vi "ultrasonic (SubVI).vi"(11 "[ESC] in":bool) -> (1 "Boolean":bool, 2 "range [centimeters] 2":sgl(slide) scale=0.0..80.0, 3 "range finder output 2":string, 4 "0, 1":i16)   [LabVIEW 2021]
uses:
  <vilib>/Instr/_visa.llb/VISA Configure Serial Port (Instr).vi
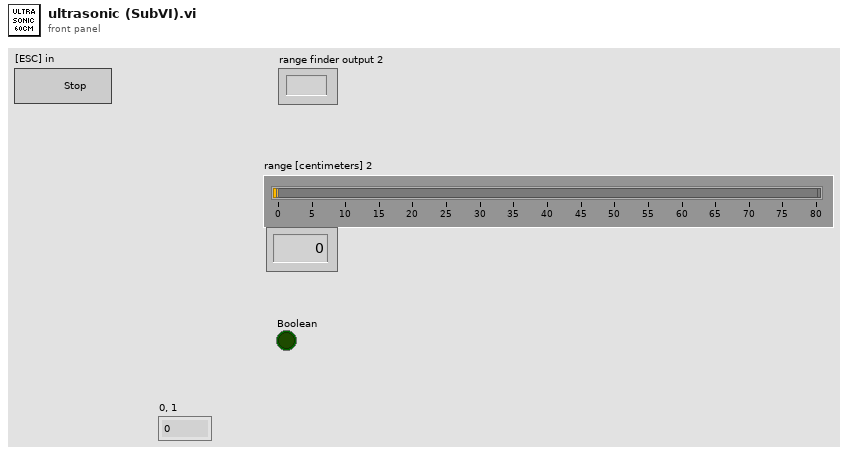
[diagram p1: front panel]
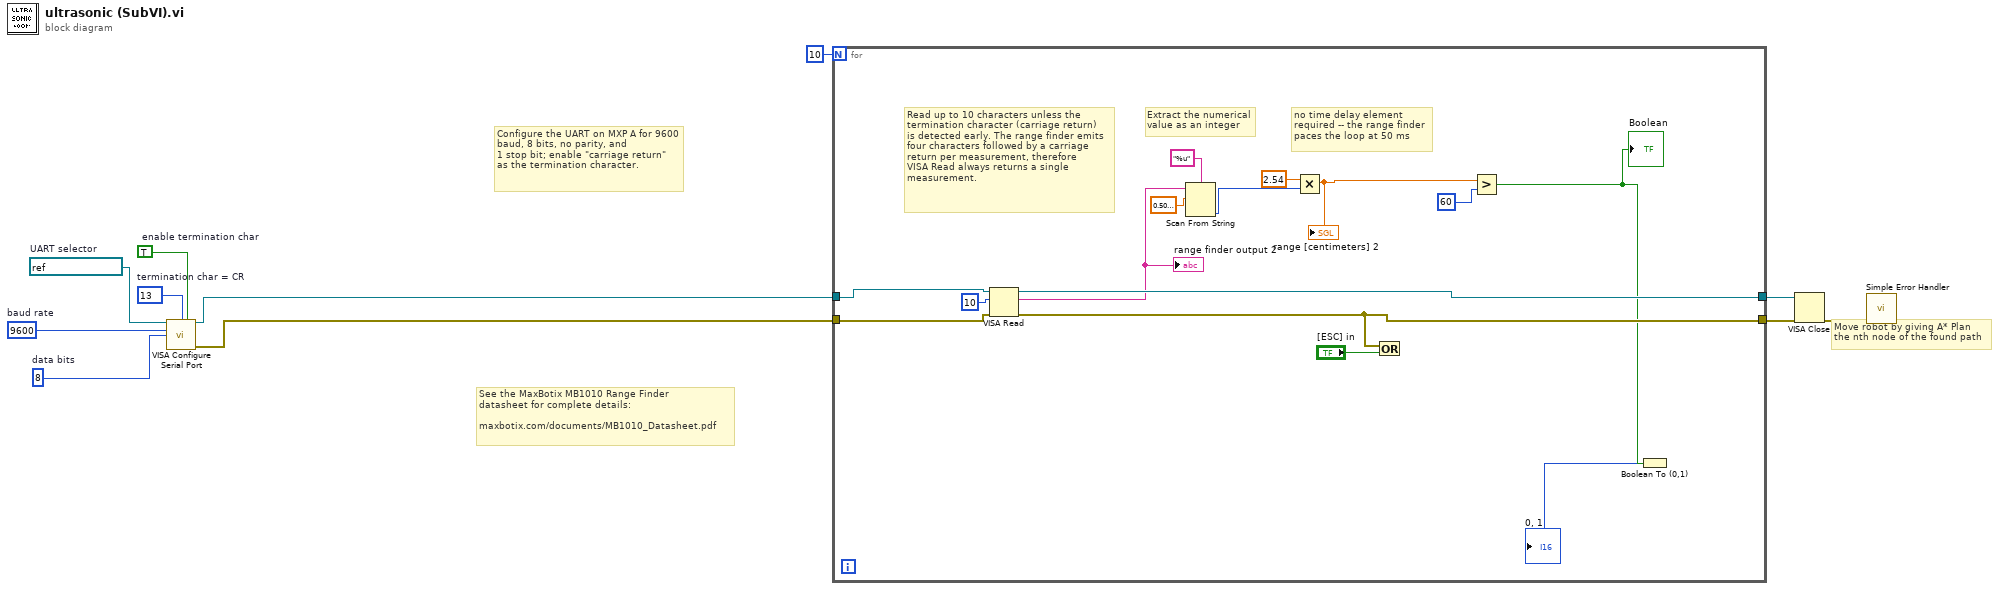
[diagram p0: block diagram]
diagram:
  w4 = u16 8  # data bits
  w5 = u32 9600  # baud rate
  w8 = refnum<visa-resource-name> "ASRL1::INSTR"  # UART selector
  w7 = u8 13  # termination char = CR
  w6 = TRUE  # enable termination char
  # "See the MaxBotix MB1010 Range Finder\ndatasheet for complete details:\n\nmaxbotix.com/documents/MB1010_Datasheet.pdf"
  # "Configure the UART on MXP A for 9600 baud, 8 bits, no parity, and\n1 stop bit; enable \"carriage return\"\nas the termination character."
  # "Move robot by giving A* Plan\nthe nth node of the found path"
  n1 = call-poly "VISA Configure Serial Port"("VISA resource name"=w8, "termination char\n(0xA = '\\n' = LF)"=w7, "Enable Termination\nChar (T)"=w6, "baud rate (9600)"=w5, "data bits (8)"=w4) -> ("VISA resource name out"=w3:refnum<visa-resource-name>, "error out"=w2:errorcluster)  [unwired: 9 in]
  n2 = for {
    N: 10 -> [_]
    tunnel: w3 -> [w24]
    tunnel: [w25] -> w9
    tunnel: w2 -> [w23]
    tunnel: [w26] -> w10
    # "Read up to 10 characters unless the \ntermination character (carriage return)\nis detected early. The range finder emits\nfour characters followed by a carriage\nreturn per measurement, therefore\nVISA Read always returns a single measurement."
    # "no time delay element\nrequired -- the range finder\npaces the loop at 50 ms"
    # "Extract the numerical\nvalue as an integer"
    n3 = VISA Read(VISA resource name=w24, byte count=u32 10, error in (no error)=w23) -> (VISA resource name out=w25:refnum<visa-resource-name>, read buffer=w18:string, error out=w26:errorcluster)  [unwired: 1 out]
    "range finder output 2" <- w18
    n4 = Scan From String "Scan From String"(format string="%u", input string=w18, initial scan location=sgl 0.51) -> (output 1=w16:u32)  [unwired: 2 in, 3 out]
    n5 = Multiply(x=2.54, y=w16) -> (x*y=w12:dbl)
    "range [centimeters] 2" <- w12
    n6 = Or(x=w26, y="[ESC] in") -> ()  [unwired: 1 out]
    n7 = Greater?(x=w12, y=60 ("x")) -> (0:w14:bool)
    "Boolean" <- w14
    n8 = Boolean To (0,1)(Boolean=w14) -> (0, 1=→"0, 1":i16)
  }
  n9 = VISA Close(VISA resource name=w9, error in (no error)=w10) -> (error out=w11:errorcluster)
  n10 = call <vilib>:"Simple Error Handler.vi"("error in (no error)"=w11) -> ()  [unwired: 4 in, 5 out]
